vi "nanostage-moving.vi"(2 "error in":errorcluster, 3 "Axes to query":string[](array[string])) -> (0 "error out":errorcluster, 1 "moving":bool)   [LabVIEW 2015]
panel:
  in  "accuracy for method 2":u8
  in  "Method":i32=1
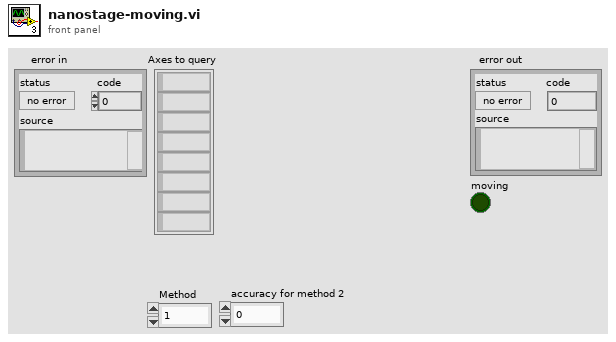
[diagram p1: front panel]
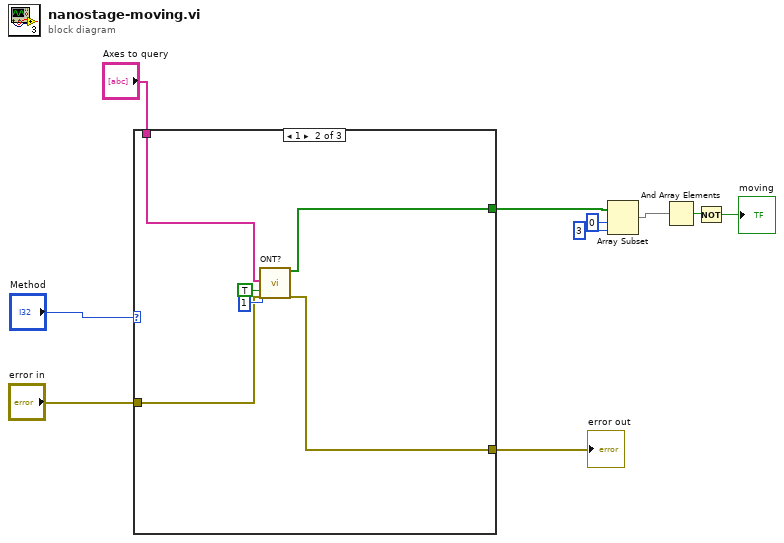
[diagram p0: block diagram]
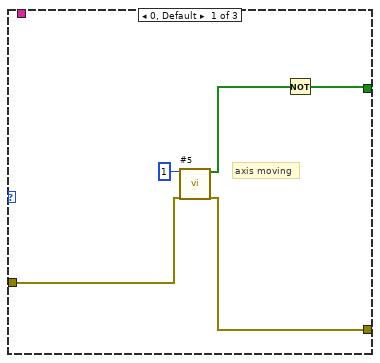
[diagram p2: hidden frame]
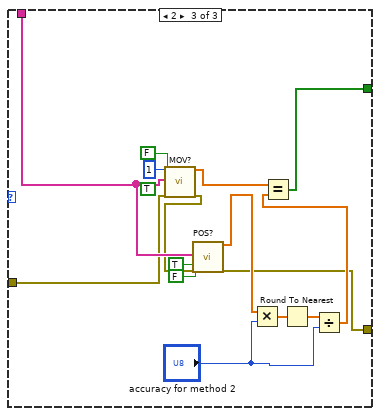
[diagram p3: hidden frame]
diagram:
  n1 = case shown="1" "Method" {
    tunnel: [w14 w20 w31] -> w7
    tunnel: "Axes to query" -> [_ w18 w35]
    tunnel: "error in" -> [w12 w17 w23]
    tunnel: [w11 w16 w22] -> w1
    frame 0, Default {
      # "axis moving"
      n2 = call "#5.vi"("System no."=1, "error in"=w12) -> ("Axis moving?"=w13:bool[], "error out"=w11:errorcluster)  [unwired: 16 in]
      n3 = Not(x=w13) -> (.not. x?=w14:bool[])
    }
    frame 1 {
      n4 = call "ONT?.vi"("System no."=1, "Axes to query"=w18, "Axis identifier?"=TRUE, "error in"=w17) -> ("Axis on target?"=w20:bool[], "error out"=w16:errorcluster)  [unwired: 14 in]
    }
    frame 2 {
      (unwired) TRUE ("Axis identifier?")
      n5 = call "MOV?.vi"("System no."=1, "Axes to query"=w35, "All axes?"=FALSE, "error in"=w23) -> ("Target position"=w32:dbl[], "error out"=w34:errorcluster)  [unwired: 14 in]
      n6 = call "POS?.vi"("Axes to query"=w35, "All axes?"=FALSE, "Axis identifier?"=TRUE, "error in"=w34) -> ("Position"=w28:dbl[], "error out"=w22:errorcluster)  [unwired: 14 in]
      n7 = Multiply(x=w28, y="accuracy for method 2") -> (x*y=w30:dbl[])
      n8 = Round To Nearest(number=w30) -> (nearest integer value=w29:dbl[])
      n9 = Divide(x=w29, y="accuracy for method 2") -> (x/y=w27:dbl[])
      n10 = Equal?(x=w32, y=w27) -> (x = y?=w31:bool[])
    }
  }
  "error out" <- w1
  n11 = Array Subset(array=w7, index=0, length=3) -> (w8:bool[])
  n12 = And Array Elements(Boolean array=w8) -> (logical AND=w6:bool)
  n13 = Not(x=w6) -> (.not. x?=→"moving":bool)
